vi "Create Enum Mapper.vi"(8 "error in":errorcluster, 9 "format string":string, 10 "RPC Message Name":string, 11 "Library item in":refnum<vi>) -> (0 "error out":errorcluster, 2 "VI out":refnum<vi>, 3 "Library item out":refnum<vi>)   [LabVIEW 2019, in "gRPC Template Creation Utility.lvlib"]
uses:
  gRPC Template Creation Utility.lvlib
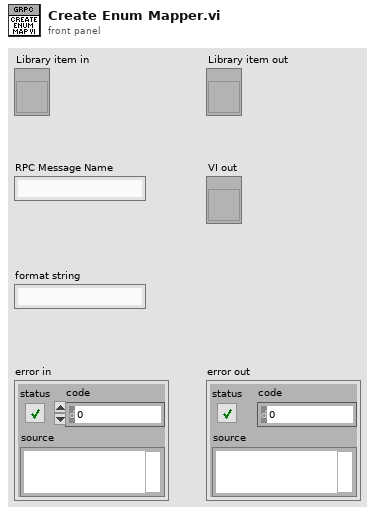
[diagram p1: front panel]
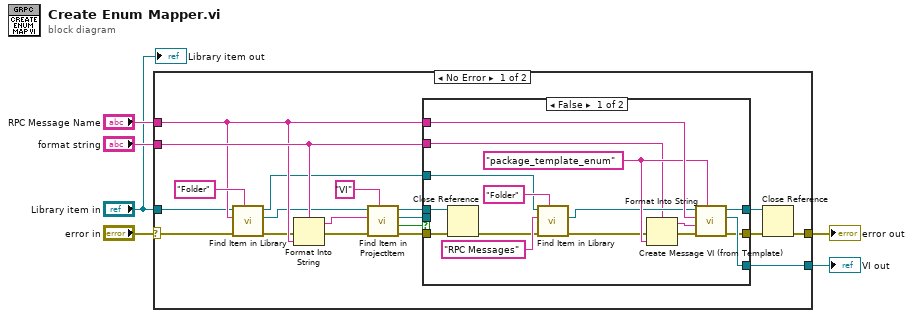
[diagram p0: block diagram]
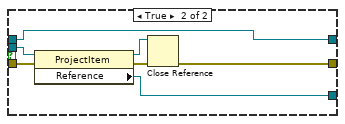
[diagram p2: hidden frame]
diagram:
  n1 = case shown="No Error" "error in" {
    selector: "error in" -> [w13 w49]
    tunnel: [w25 _] -> w6
    tunnel: [w7 w49] -> w5
    tunnel: "RPC Message Name" -> [w15 _]
    tunnel: "format string" -> [w18 _]
    tunnel: "Library item in" -> [w14 _]
    frame No Error {
      n2 = call "Find Item in Library.vi"("Item Type"="Folder", "error in (no error)"=w13, "Item Name"=w15, "Library item in"=w14) -> ("error out"=w12:errorcluster, "Project Item (Library Item)"=w10:refnum<vi>, "Library item out"=w11:refnum<vi>)  [unwired: 4 in, 1 out]
      n3 = Format Into String(format string=w18, error in=w12, w15) -> (resulting string=w19:string, error out=w17:errorcluster)  [unwired: 1 in]
      n4 = call "Find Item in ProjectItem.vi"("Item Type"="VI", "error in (no error)"=w17, "Name"=w19, "ProjectItem in"=w10) -> ("error out"=w21:errorcluster, "Found ?"=w22:bool, "Item Refnum out"=w20:refnum<vi>, "ProjectItem out"=w23:refnum<vi>)  [unwired: 4 in]
      n5 = case shown="False" w22 {
        tunnel: [w39 w47] -> w25
        tunnel: [w40 w46] -> w9
        tunnel: w21 -> [w28 w43]
        tunnel: [w38 w42] -> w8
        tunnel: w23 -> [w26 w46]
        tunnel: w20 -> [_ w48]
        tunnel: w15 -> [w41 _]
        tunnel: w18 -> [w29 _]
        tunnel: w11 -> [w31 _]
        frame False {
          w37 = "package_template_enum" ("replace string in template")
          n6 = Close Reference(reference=w26, error in (no error)=w28) -> (error out=w27:errorcluster)
          n7 = call "Find Item in Library.vi"("Item Type"="Folder", "error in (no error)"=w27, "Item Name"="RPC Messages", "Library item in"=w31) -> ("error out"=w30:errorcluster, "Project Item (Library Item)"=w32:refnum<vi>)  [unwired: 4 in, 2 out]
          n8 = Format Into String(format string=w29, error in=w30, w37) -> (resulting string=w36:string, error out=w35:errorcluster)  [unwired: 1 in]
          n9 = call "Create Message VI (from Template).vi"("replace string in template"=w37, "error in (no error)"=w35, "template VI name"=w36, "RPC Message Name"=w41, "RPC Messages Folder (ProjectItem) in"=w32) -> ("error out"=w38:errorcluster, "Getter VI out"=w39:refnum<vi>, "RPC Messages Folder (ProjectItem) out"=w40:refnum<vi>)  [unwired: 3 in, 1 out]
        }
        frame True {
          n10 = property class="ProjectItem"(reference=w48, error in=w43) -> (reference out=w44:refnum<vi>, error out=w45:errorcluster, "Reference"=w47:refnum<vi>)
          n11 = Close Reference(reference=w44, error in (no error)=w45) -> (error out=w42:errorcluster)
        }
      }
      n12 = Close Reference(reference=w9, error in (no error)=w8) -> (error out=w7:errorcluster)
    }
    frame Error {
    }
  }
  "error out" <- w5
  "VI out" <- w6
  "Library item out" <- "Library item in"
